vi "WiiBalanceBoard_Get_Sensors.vi"(5 "hWiimoteHandle in":u32, 6 "Wii Balance Board Zeros":T2, 7 "error in":errorcluster) -> (0 "hWiimoteHandle out":u32, 1 "Button":bool, 2 "Wii Balance Board Sensors":T1, 3 "error out":errorcluster, 4 "pReportBuffer out":u8[](array[numeric]) format="%02d")   [LabVIEW 2010]
doc: "CETPD\nCalculates the CG of the Board (X,Y) adjusting the actual value of the sensors with the Zero Calibration.\nToo returns if the button is pressed."
uses:
  Wiimote Reporting Mode.ctl
panel:
  out "Suma":dbl
  out "X":dbl
  out "Y":dbl
  out "Left-bottom":i16
  out "Left-top":i16
  out "Right-bottom":i16
  out "Right-top":i16
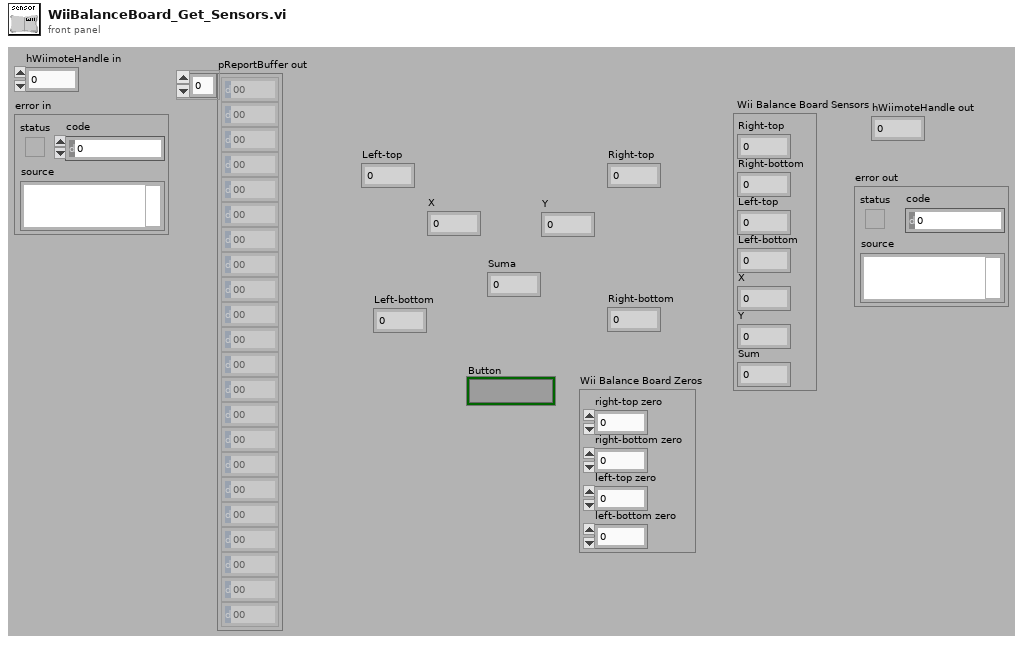
[diagram p1: front panel]
types:
  T1 = cluster{"Right-top":i16, "Right-bottom":i16, "Left-top":i16, "Left-bottom":i16, "X":dbl, "Y":dbl, "Sum":dbl}
  T2 = cluster{"right-top zero":i16, "right-bottom zero":i16, "left-top zero":i16, "left-bottom zero":i16}
  T3 = typedef "Wiimote Reporting Mode.ctl" = u8
  T4 = typedef "Wiimote Buttons.ctl" = cluster{"D-Pad Left":bool, "D-Pad Right":bool, "D-Pad Down":bool, "D-Pad Up":bool, "Plus":bool, "Two":bool, "One":bool, "B":bool, "A":bool, "Minus":bool, "Home":bool}
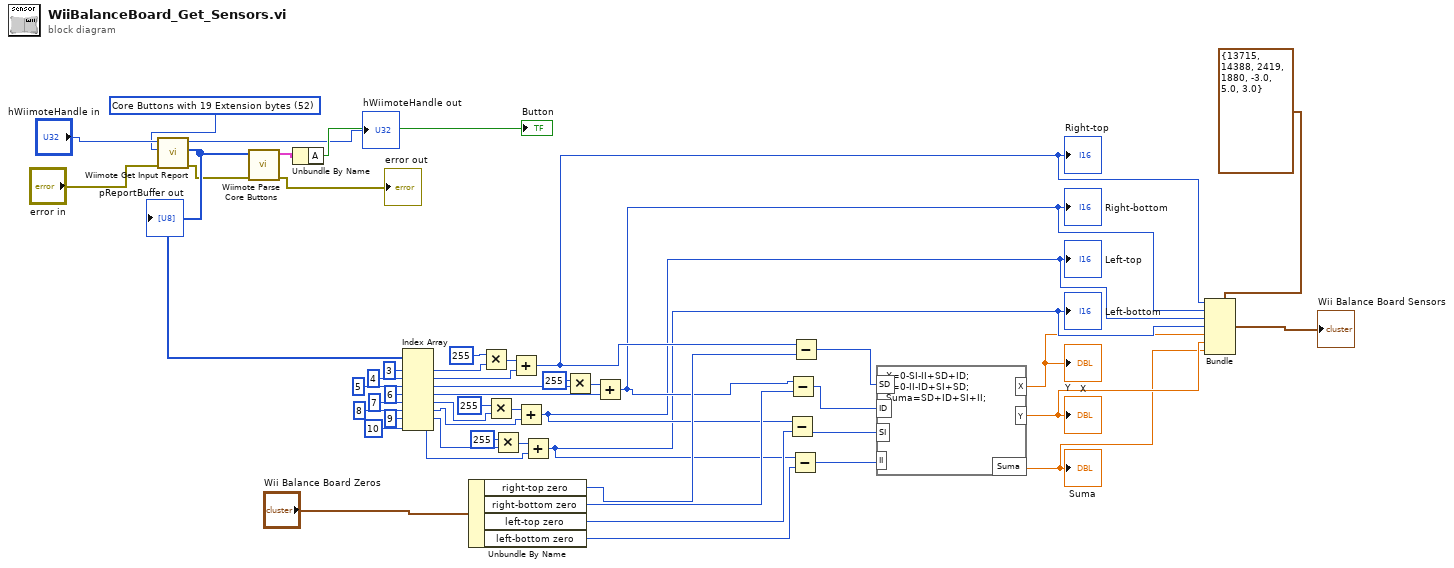
[diagram p0: block diagram]
diagram:
  w10 = T3 52 items=["Core Buttons"=48, "Core Buttons and Accelerometer"=49, "Core Buttons with 8 Extension bytes"=50, "Core Buttons and Accelerometer with 12 IR bytes"=51, "Core Buttons with 19 Extension bytes"=52, "Core Buttons and Accelerometer with 16 Extension Bytes"=53, "Core Buttons with 10 IR bytes and 9 Extension Bytes"=54, "Core Buttons and Accelerometer with 10 IR bytes and 6 Extension Bytes"=55] ("Reporting Mode")
  n1 = call "Wiimote Get Input Report.vi"("error in"="error in", "bInputReport"=w10, "hWiimoteHandle in"="hWiimoteHandle in") -> ("error out"=w11:errorcluster, "pReportBuffer out"=w16:u8[], "hWiimoteHandle out"=→"hWiimoteHandle out":u32)  [unwired: 6 in]
  "pReportBuffer out" <- w16
  n2 = call "Wiimote Parse Core Buttons.vi"("error in"=w11, "pReportBuffer in"=w16) -> ("error out"=→"error out":errorcluster, "Wiimote Buttons out"=w14:T4)  [unwired: 8 in]
  n3 = Unbundle By Name(w14) -> ("A"=→"Button":bool)
  n4 = Index Array(array=w16, index #1=3 ("index"), index #2=4 ("index"), index #3=5 ("index"), index #4=6 ("index"), index #5=7 ("index"), index #6=8 ("index"), index #7=9 ("index"), index #8=10 ("index")) -> (element #1=w30:u8, element #2=w26:u8, element #3=w31:u8, element #4=w28:u8, element #5=w35:u8, element #6=w34:u8, element #7=w39:u8, element #8=w40:u8)
  n5 = Unbundle By Name("Wii Balance Board Zeros") -> ("right-top zero"=w48:i16, "right-bottom zero"=w49:i16, "left-top zero"=w50:i16, "left-bottom zero"=w51:i16)
  n6 = Multiply(x=i16 255 ("y"), y=w30) -> (x*y=w25:i16)
  n7 = Multiply(x=i16 255 ("y"), y=w35) -> (x*y=w33:i16)
  n8 = Multiply(x=i16 255 ("y"), y=w39) -> (x*y=w37:i16)
  n9 = Add(x=w25, y=w26) -> (x+y=w9:i16)
  "Right-top" <- w9
  n10 = Add(x=w33, y=w34) -> (x+y=w7:i16)
  "Left-top" <- w7
  n11 = Add(x=w37, y=w40) -> (x+y=w6:i16)
  "Left-bottom" <- w6
  n12 = Multiply(x=i16 255 ("y"), y=w31) -> (x*y=w27:i16)
  n13 = Add(x=w27, y=w28) -> (x+y=w8:i16)
  "Right-bottom" <- w8
  n14 = Subtract(x=w7, y=w50) -> (x-y=w43:i16)
  n15 = Subtract(x=w8, y=w49) -> (x-y=w42:i16)
  n16 = Subtract(x=w6, y=w51) -> (x-y=w44:i16)
  n17 = Subtract(x=w9, y=w48) -> (x-y=w41:i16)
  n18 = formula code="X=0-SI-II+SD+ID;\nY=0-II-ID+SI+SD;\nSuma=SD+ID+SI+II;"("SD"=w41, "ID"=w42, "SI"=w43, "II"=w44) -> ("X"=w5:dbl, "Y"=w4:dbl, "Suma"=w3:dbl)
  "Y" <- w4
  "X" <- w5
  "Suma" <- w3
  n19 = Bundle(cluster=T1 {"Right-top"=13715, "Right-bottom"=14388, "Left-top"=2419, "Left-bottom"=1880, "X"=-3.0, "Y"=5.0, "Sum"=3.0}, "Right-top"=w9, "Right-bottom"=w8, "Left-top"=w7, "Left-bottom"=w6, "X"=w5, "Y"=w4, "Sum"=w3) -> (→"Wii Balance Board Sensors":T1)
